vi "Data.vi"(8 "error in (no error)":errorcluster, 10 "Data":string[][](array[string])) -> (0 "error out":errorcluster)   [LabVIEW 2018, in "MQTT Messages.lvlib"]
uses:
  MQTT Messages.lvlib
  MQTT_Singleton/MQTT_Singleton.lvlib
panel:
  out "JSON string":string
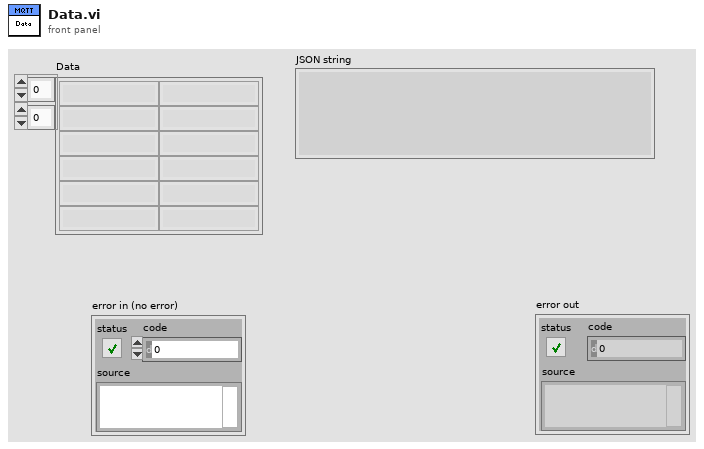
[diagram p1: front panel]
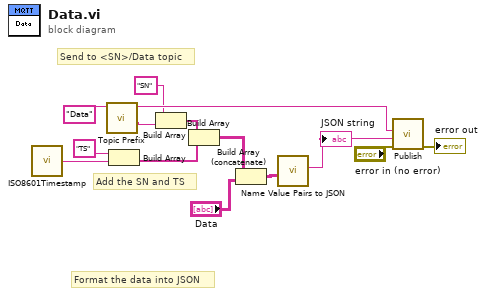
[diagram p0: block diagram]
diagram:
  # "Add the SN and TS"
  # "Format the data into JSON"
  # "Send to <SN>/Data topic"
  n1 = call "ISO8601Timestamp.vi"() -> ("date/time string"=w8:string)  [unwired: 5 in]
  n2 = call "Topic Prefix.vi"("Topic"="Data" ("string")) -> ("SN"=w6:string, "Topic"=w13:string)  [unwired: 9 in]
  n3 = Build Array("TS" ("element"), w8) -> (w4:string[])
  n4 = Build Array("SN" ("element"), w6) -> (w5:string[])
  n5 = Build Array(w5, w4) -> (w3:string[][])
  n6 = Build Array (concatenate)(w3, "Data") -> (w1:string[][])
  n7 = call "Name Value Pairs to JSON.vi"("Message"=w1) -> ("JSON string"=w10:string)  [unwired: 10 in]
  "JSON string" <- w10
  n8 = call "Publish.vi"("error in (no error)"="error in (no error)", "Message"=w10, "Topic"=w13) -> ("error out"=→"error out":errorcluster)  [unwired: 8 in]
